vi "ke37xx Configure Totalizer Channel Mode.vi"(8 "error in (no error)":errorcluster, 9 "Mode (Rising Edge TTL)":T1(ring)=enum."Rising Edge TTL", 10 "Totalizer Channels":string, 11 "VISA Resource Name":refnum<visa-resource-name>) -> (0 "error out":errorcluster, 3 "VISA Resource Name Out":refnum<visa-resource-name>)   [LabVIEW 2009, in "Keithley 3700 Series.lvlib"]
doc: "This VI configures the Totalizer channel mode and sets how its triggered."
uses:
  <instrlib>/Keithley 3706/Keithley 3700 Series.lvlib
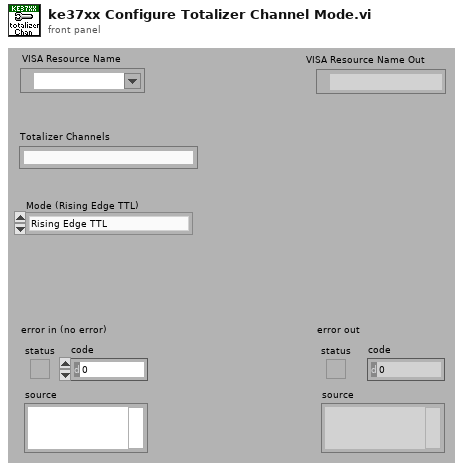
[diagram p1: front panel]
types:
  T1 = enum8{"Rising Edge", "Falling Edge", "Rising Edge TTL", "Falling Edge TTL", "Rising Edge Read Reset", "Falling Edge Read Reset", "Rising Edge TTL Edge Read Reset", "Falling Edge TTL Edge Read Reset"}
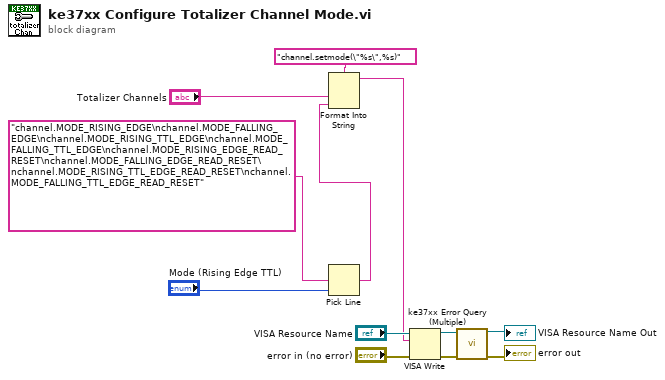
[diagram p0: block diagram]
diagram:
  n1 = Pick Line(multi-line string="channel.MODE_RISING_EDGE\nchannel.MODE_FALLING_EDGE\nchannel.MODE_RISING_TTL_EDGE\nchannel.MODE_FALLING_TTL_EDGE\nchannel.MODE_RISING_EDGE_READ_RESET\nchannel.MODE_FALLING_EDGE_READ_RESET\nchannel.MODE_RISING_TTL_EDGE_READ_RESET\nchannel.MODE_FALLING_TTL_EDGE_READ_RESET", line index="Mode (Rising Edge TTL)") -> (output string=w3:string)  [unwired: 1 out]
  n2 = Format Into String(format string="channel.setmode(\"%s\",%s)", "Totalizer Channels", w3) -> (resulting string=w7:string)  [unwired: 2 in, 1 out]
  n3 = VISA Write(VISA resource name="VISA Resource Name", write buffer=w7, error in (no error)="error in (no error)") -> (VISA resource name out=w6:refnum<visa-resource-name>, error out=w5:errorcluster)  [unwired: 1 out]
  n4 = call <instrlib>:"ke37xx Error Query (Multiple).vi"("VISA resource name"=w6, "error in (no error)"=w5) -> ("VISA resource name out"=→"VISA Resource Name Out":refnum<visa-resource-name>, "error out"=→"error out":errorcluster)  [unwired: 12 out]
